vi "MCUConfigMessage.vi"(8 "AScanFrequency":dbl, 10 "ScanningMode":T1, 11 "OctType":T2) -> (3 "MCUConfigMessage":string)   [LabVIEW 2019]
uses:
  OCTTypeTypeDef.ctl
  ScanningModeTypeDef.ctl
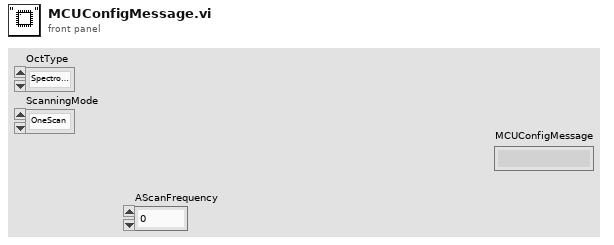
[diagram p1: front panel]
types:
  T1 = typedef "ScanningModeTypeDef.ctl" = enum16{"OneScan", "ContinuousScan"}
  T2 = typedef "OCTTypeTypeDef.ctl" = enum16{"Spectrometer OCT", "SSOCT"}
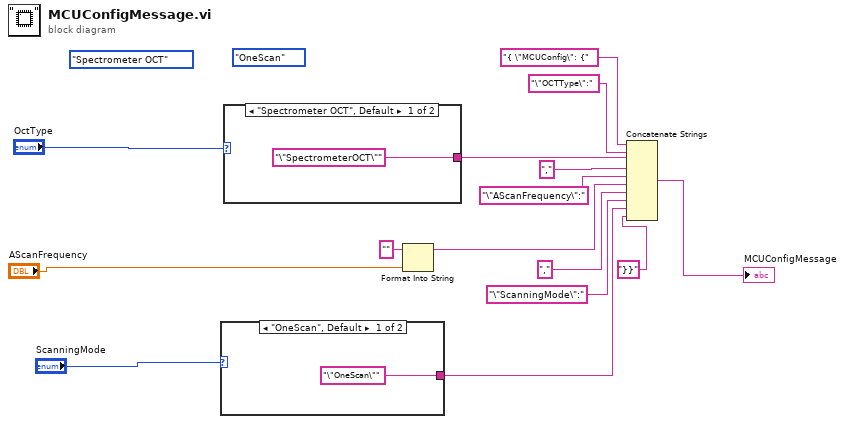
[diagram p0: block diagram]
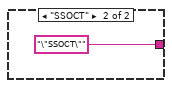
[diagram p2: hidden frame]
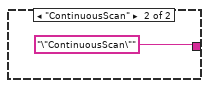
[diagram p3: hidden frame]
diagram:
  (unwired) ScanningModeTypeDef."OneScan"
  (unwired) OCTTypeTypeDef."Spectrometer OCT"
  n1 = case shown="\"OneScan\", Default" "ScanningMode" {
    tunnel: ["\"OneScan\"" ("MCUConfigMessage") "\"ContinuousScan\"" ("MCUConfigMessage")] -> w1
    frame "OneScan", Default {
    }
    frame "ContinuousScan" {
    }
  }
  n2 = case shown="\"Spectrometer OCT\", Default" "OctType" {
    tunnel: ["\"SpectrometerOCT\"" ("MCUConfigMessage") "\"SSOCT\"" ("MCUConfigMessage")] -> w12
    frame "Spectrometer OCT", Default {
    }
    frame "SSOCT" {
    }
  }
  n3 = Format Into String(initial string="", "AScanFrequency") -> (resulting string=w7:string)  [unwired: 2 in, 1 out]
  n4 = Concatenate Strings("{ \"MCUConfig\": {" ("MCUConfigMessage"), "\"OCTType\":" ("MCUConfigMessage"), w12, "," ("string"), "\"AScanFrequency\":" ("string"), w7, "," ("string"), "\"ScanningMode\":" ("string"), w1, "}}" ("string")) -> (→"MCUConfigMessage":string)
